vi "StripQuality.vi"(0 "No of entries":i32, 1 "Capacitance Data Array":dbl[](array[numeric]), 2 "Channel No. Array":dbl[](array[numeric]), 3 "Pinhole flag array in":dbl[](array[numeric]), 4 "Resistance data array":dbl[](array[numeric]), 5 "Thresholds":T1, 6 "Defect Flag array IN":i32[][](array[numeric])) -> (7 "Defect code":i32, 8 "Strip Quality Data":T2 {"pass Rate in %" format="%.2f"})   [LabVIEW 2018]
panel:
  # "Current [nA]:"
  # "Capacitance [pF]:"
  # "Resistance [MW]:"
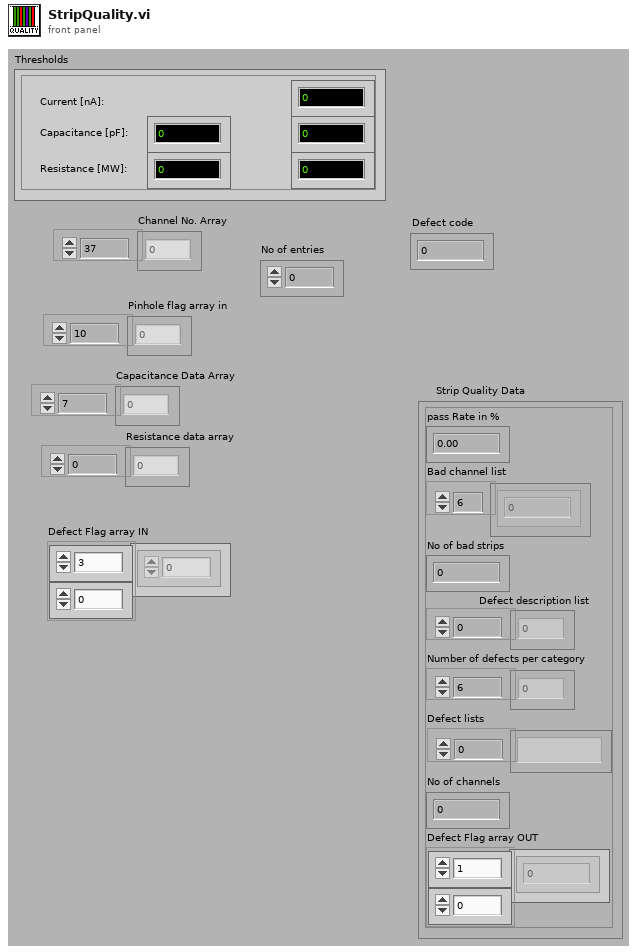
[diagram p1: front panel]
types:
  T1 = cluster{"Current [nA]":dbl, "Cap_Lo":dbl, "Cap_Hi":dbl, "Res_Hi":dbl, "Res_Lo":dbl}
  T2 = cluster{"pass Rate in %":dbl, "Bad channel list":i32[], "No of bad strips":i32, "Defect description list":i32[], "Number of defects per category":i32[], "Defect lists":string[], "No of channels":i32, "Defect Flag array OUT":i32[][]}
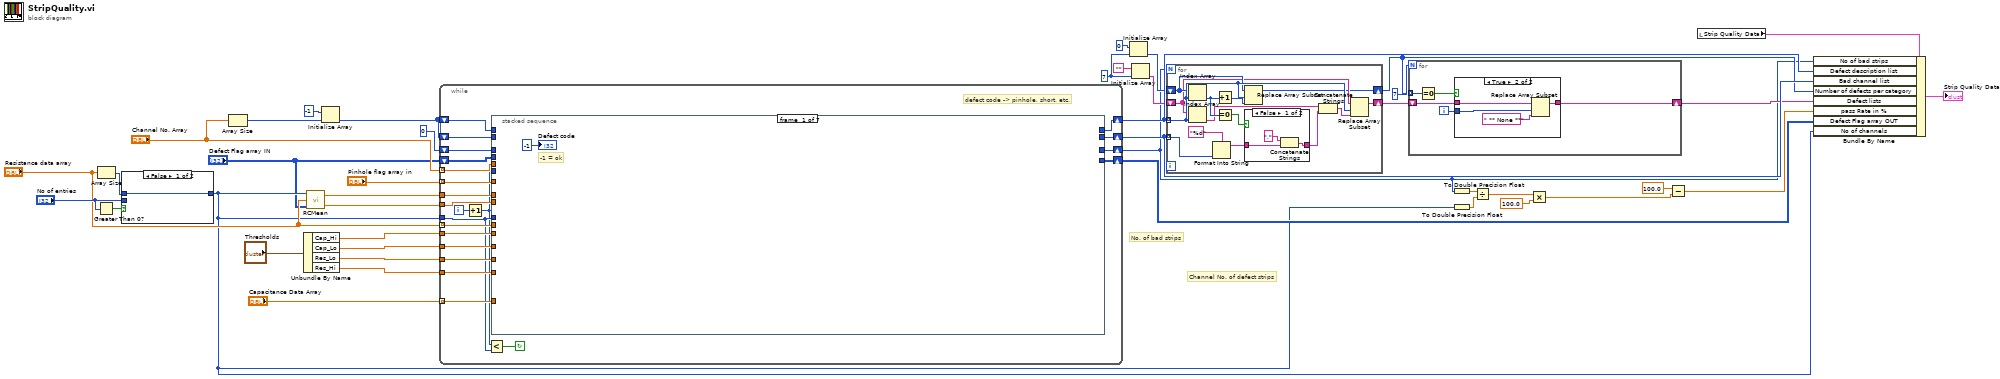
[diagram p0: block diagram]
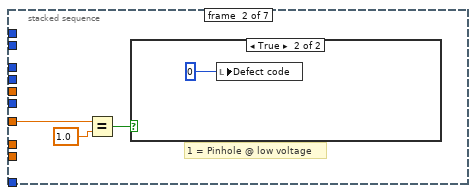
[diagram p2: hidden frame]
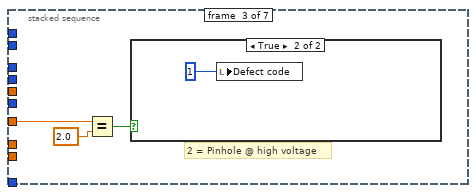
[diagram p4: hidden frame]
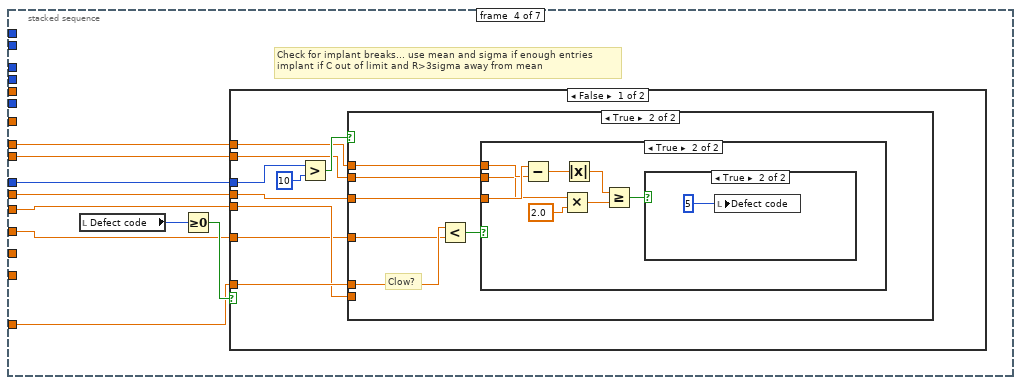
[diagram p6: hidden frame]
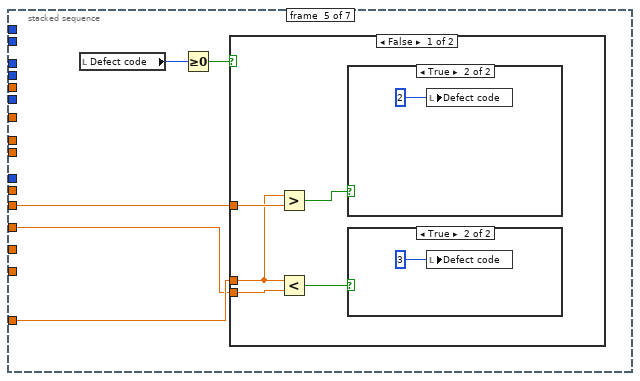
[diagram p11: hidden frame]
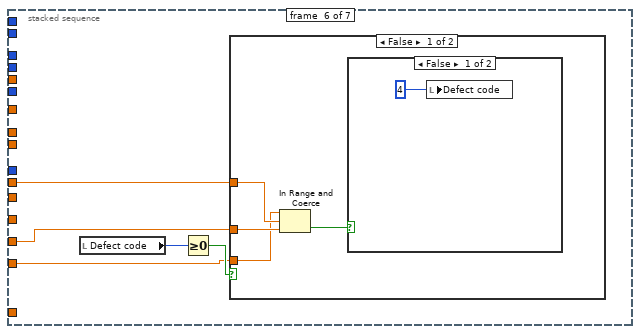
[diagram p15: hidden frame]
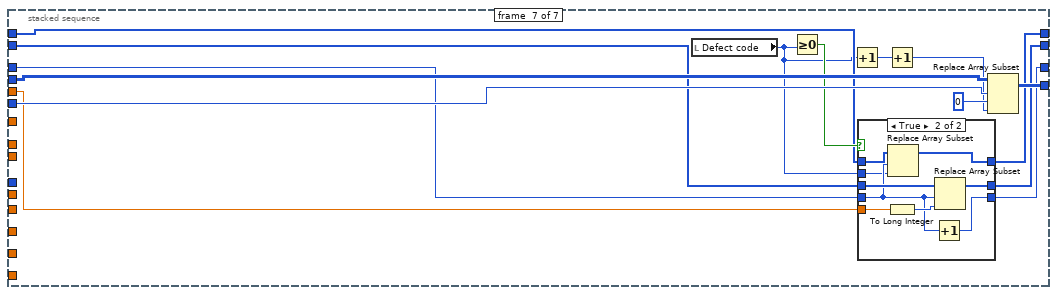
[diagram p18: hidden frame]
diagram:
  w26 = 7 ("Dimension Size")
  # "No. of bad strips"
  # "Channel No. of defect strips"
  n1 = Greater Than 0?(x="No of entries") -> (x > 0?=w8:bool)
  n2 = Array Size(array="Resistance data array") -> (size(s)=w5:i32)
  n3 = case shown="False" w8 {
    tunnel: "No of entries" -> [_ w44]
    tunnel: [w43 w44] -> w4
    tunnel: w5 -> [w43 _]
    frame False {
    }
    frame True {
    }
  }
  n4 = Array Size(array="Channel No. Array") -> (size(s)=w34:i32)
  n5 = Unbundle By Name("Thresholds") -> ("Cap_Hi"=w1:dbl, "Cap_Lo"=w40:dbl, "Res_Lo"=w37:dbl, "Res_Hi"=w36:dbl)
  n6 = call "RCMean.vi"("Defect Flag array IN"="Defect Flag array IN", "data array in"="Resistance data array", "No of strips"=w4) -> ("standard deviation"=w38:dbl, "mean"=w39:dbl)
  n7 = Initialize Array(-1, w34) -> (w32:i32[])
  n8 = while {
    shift-left: 0 -> [w50]
    shift-right: [w49] -> w16
    shift-left: w32 -> [w53]
    shift-right: [w48] -> w28
    shift-left: w32 -> [w54]
    shift-right: [w51] -> w27
    shift-left: "Defect Flag array IN" -> [w56]
    shift-right: [w55] -> w17
    tunnel: w36 -> [w57]
    tunnel: w37 -> [w58]
    tunnel: w38 -> [w59]
    tunnel: w39 -> [w60]
    tunnel: "Resistance data array" -> [w61] mode=indexing
    tunnel: w40 -> [w62]
    tunnel: w1 -> [w63]
    tunnel: "Capacitance Data Array" -> [w64] mode=indexing
    tunnel: "Channel No. Array" -> [w52] mode=indexing
    tunnel: "Pinhole flag array in" -> [w65] mode=indexing
    tunnel: w4 -> [w47]
    i -> [w46]
    stop <- w66 continue-if-true
    # "defect code -> pinhole, short, etc."
    n9 = Increment(x=w46) -> (x+1=w45:i32)
    n10 = Less?(x=w45, y=w47) -> (x < y?=w66:bool)
    n11 = stacked-sequence {
      tunnel: w65 -> [_ w70 w74 _ _ _ _]
      tunnel: w47 -> [_ _ _ w82 _ _ _]
      tunnel: w64 -> [_ _ _ w81 w111 _ _]
      tunnel: w63 -> [_ _ _ w80 w110 _ _]
      tunnel: w62 -> [_ _ _ w79 w109 _ _]
      tunnel: w61 -> [_ _ _ w78 _ w123 _]
      tunnel: w60 -> [_ _ _ w77 _ _ _]
      tunnel: w59 -> [_ _ _ w76 _ _ _]
      tunnel: w58 -> [_ _ _ _ _ w122 _]
      tunnel: w57 -> [_ _ _ _ _ w121 _]
      tunnel: w56 -> [_ _ _ _ _ _ w145]
      tunnel: w45 -> [_ _ _ _ _ _ w144]
      tunnel: [_ _ _ _ _ _ w142] -> w55
      tunnel: w54 -> [_ _ _ _ _ _ w141]
      tunnel: w53 -> [_ _ _ _ _ _ w137]
      tunnel: w52 -> [_ _ _ _ _ _ w140]
      tunnel: [_ _ _ _ _ _ w139] -> w51
      tunnel: w50 -> [_ _ _ _ _ _ w136]
      tunnel: [_ _ _ _ _ _ w135] -> w49
      tunnel: [_ _ _ _ _ _ w134] -> w48
      frame #0 {
        # "-1 = ok"
        "Defect code" <- -1 ("Defect code")
      }
      frame #1 {
        # "1 = Pinhole @ low voltage"
        n12 = Equal?(x=w70, y=1.0) -> (x = y?=w68:bool)
        n13 = case shown="True" w68 {
          frame False {
          }
          frame True {
            n14 = local write "Defect code"(0 ("Defect code")) -> ()
          }
        }
      }
      frame #2 {
        # "2 = Pinhole @ high voltage"
        n15 = Equal?(x=w74, y=2.0) -> (x = y?=w72:bool)
        n16 = case shown="True" w72 {
          frame False {
          }
          frame True {
            n17 = local write "Defect code"(1 ("Defect code")) -> ()
          }
        }
      }
      frame #3 {
        # "Check for implant breaks... use mean and sigma if enough entries\nimplant if C out of limit and R>3sigma away from mean"
        n18 = local read "Defect code"() -> (w84:i32)
        n19 = Greater Or Equal To 0?(x=w84) -> (x >= 0?=w83:bool)
        n20 = case shown="False" w83 {
          tunnel: w82 -> [w93 _]
          tunnel: w81 -> [w90 _]
          tunnel: w80 -> [w89 _]
          tunnel: w79 -> [w88 _]
          tunnel: w78 -> [w87 _]
          tunnel: w77 -> [w86 _]
          tunnel: w76 -> [w85 _]
          frame False {
            n21 = Greater?(x=w93, y=10) -> (0:w91:bool)
            n22 = case shown="True" w91 {
              tunnel: w90 -> [_ w99]
              tunnel: w89 -> [_ _]
              tunnel: w88 -> [_ w98]
              tunnel: w87 -> [_ w96]
              tunnel: w86 -> [_ w95]
              tunnel: w85 -> [_ w94]
              frame False {
              }
              frame True {
                # "Clow?"
                n23 = Less?(x=w99, y=w98) -> (x < y?=w97:bool)
                n24 = case shown="True" w97 {
                  tunnel: w96 -> [_ w107]
                  tunnel: w95 -> [_ w106]
                  tunnel: w94 -> [_ w104]
                  frame False {
                  }
                  frame True {
                    n25 = Subtract(x=w107, y=w106) -> (x-y=w105:dbl)
                    n26 = Multiply(x=w104, y=2.0) -> (x*y=w101:dbl)
                    n27 = Absolute Value(x=w105) -> (abs(x)=w102:dbl)
                    n28 = Greater Or Equal?(x=w102, y=w101) -> (x >= y?=w100:bool)
                    n29 = case shown="True" w100 {
                      frame False {
                      }
                      frame True {
                        n30 = local write "Defect code"(5 ("Defect code")) -> ()
                      }
                    }
                  }
                }
              }
            }
          }
          frame True {
          }
        }
      }
      frame #4 {
        n31 = local read "Defect code"() -> (w113:i32)
        n32 = Greater Or Equal To 0?(x=w113) -> (x >= 0?=w112:bool)
        n33 = case shown="False" w112 {
          tunnel: w111 -> [w116 _]
          tunnel: w110 -> [w118 _]
          tunnel: w109 -> [w115 _]
          frame False {
            n34 = Greater?(x=w116, y=w118) -> (0:w117:bool)
            n35 = Less?(x=w116, y=w115) -> (x < y?=w114:bool)
            n36 = case shown="True" w117 {
              frame False {
              }
              frame True {
                n37 = local write "Defect code"(2 ("Defect code")) -> ()
              }
            }
            n38 = case shown="True" w114 {
              frame False {
              }
              frame True {
                n39 = local write "Defect code"(3 ("Defect code")) -> ()
              }
            }
          }
          frame True {
          }
        }
      }
      frame #5 {
        n40 = local read "Defect code"() -> (w125:i32)
        n41 = Greater Or Equal To 0?(x=w125) -> (x >= 0?=w124:bool)
        n42 = case shown="False" w124 {
          tunnel: w123 -> [w129 _]
          tunnel: w122 -> [w128 _]
          tunnel: w121 -> [w127 _]
          frame False {
            n43 = In Range and Coerce(upper limit=w127, x=w129, lower limit=w128) -> (In Range?=w126:bool)  [unwired: 1 out]
            n44 = case shown="False" w126 {
              frame False {
                n45 = local write "Defect code"(4 ("Defect code")) -> ()
              }
              frame True {
              }
            }
          }
          frame True {
          }
        }
      }
      frame #6 {
        n46 = local read "Defect code"() -> (w131:i32)
        n47 = Greater Or Equal To 0?(x=w131) -> (x >= 0?=w138:bool)
        n48 = Increment(x=w131) -> (x+1=w132:i32)
        n49 = case shown="True" w138 {
          tunnel: w141 -> [w148 w157]
          tunnel: w140 -> [_ w155]
          tunnel: [w148 w154] -> w139
          tunnel: w137 -> [w147 w153]
          tunnel: w136 -> [w146 w150]
          tunnel: [w146 w152] -> w135
          tunnel: [w147 w151] -> w134
          tunnel: w131 -> [_ w149]
          frame False {
          }
          frame True {
            n50 = To Long Integer(number=w155) -> (32bit integer=w156:i32)
            n51 = Replace Array Subset(array=w153, new element=w149, index=w150) -> (w151:i32[])
            n52 = Increment(x=w150) -> (x+1=w152:i32)
            n53 = Replace Array Subset(array=w157, new element=w156, index=w150) -> (w154:i32[])
          }
        }
        n54 = Increment(x=w132) -> (x+1=w133:i32)
        n55 = Replace Array Subset(array=w145, new element=w133, index (row)=w144, index (col)=0 ("Index")) -> (w142:i32[][])
      }
    }
  }
  n56 = Initialize Array(0, w26) -> (w24:i32[])
  n57 = Initialize Array("", w26) -> (w23:string[])
  n58 = for {
    N: w16 -> [_]
    tunnel: w28 -> [w162] mode=indexing
    tunnel: w27 -> [w167] mode=indexing
    shift-right: [w159] -> w21
    shift-left: w24 -> [w161]
    shift-right: [w158] -> w20
    shift-left: w23 -> [w160]
    n59 = Index Array(array=w161, index=w162) -> (element=w170:i32)
    n60 = Index Array(array=w160, index=w162) -> (element=w165:string)
    n61 = Format Into String(format string="%d" ("Format String"), w167) -> (resulting string=w166:string)  [unwired: 2 in, 1 out]
    n62 = Increment(x=w170) -> (x+1=w171:i32)
    n63 = Equal To 0?(x=w170) -> (x = 0?=w169:bool)
    n64 = Replace Array Subset(array=w161, new element=w171, index=w162) -> (w159:i32[])
    n65 = case shown="False" w169 {
      tunnel: w166 -> [w172 w175]
      tunnel: [w174 w175] -> w164
      frame False {
        n66 = Concatenate Strings(",", w172) -> (w174:string)
      }
      frame True {
      }
    }
    n67 = Concatenate Strings(w165, w164) -> (w163:string)
    n68 = Replace Array Subset(array=w160, new element=w163, index=w162) -> (w158:string[])
  }
  n69 = for {
    N: 7 -> [_]
    tunnel: w21 -> [w180] mode=indexing
    shift-right: [w176] -> w19
    shift-left: w20 -> [w178]
    i -> [w177]
    n70 = Equal To 0?(x=w180) -> (x = 0?=w179:bool)
    n71 = case shown="True" w179 {
      tunnel: w178 -> [w181 w185]
      tunnel: w177 -> [_ w183]
      tunnel: [w181 w182] -> w176
      frame False {
      }
      frame True {
        n72 = Replace Array Subset(array=w185, new element=" ** None **" ("Element Data"), index=w183) -> (w182:string[])
      }
    }
  }
  n73 = To Double Precision Float(number=w16) -> (double precision float=w15:dbl)
  n74 = To Double Precision Float(number=w4) -> (double precision float=w14:dbl)
  n75 = Divide(x=w15, y=w14) -> (x/y=w13:dbl)
  n76 = Multiply(x=w13, y=100.0) -> (x*y=w10:dbl)
  n77 = Subtract(x=100.0, y=w10) -> (x-y=w9:dbl)
  n78 = local read "Strip Quality Data"() -> (w30:T2)
  n79 = Bundle By Name(cluster=w30, "No of bad strips"=w16, "Defect description list"=w28, "Bad channel list"=w27, "Number of defects per category"=w21, "Defect lists"=w19, "pass Rate in %"=w9, "Defect Flag array OUT"=w17, "No of channels"=w4) -> (→"Strip Quality Data":T2)
